vi "SetXL_CellValues_2D_Dbl.vi"(0 "Refnum Cluster In":T1, 5 "Start":cluster{"Column":i32, "Row":i32}, 9 "data":dbl[][](array[numeric]), 11 "error in":errorcluster) -> (4 "Refnum Cluster Out":T1, 15 "error out":errorcluster)   [LabVIEW 2017, in "excel_configuration.lvlib"]
uses:
  excel_configuration.lvlib
  858a33e0-4cb3-45c4-8fa4-0a07d001454b.vi
  <vilib>/Utility/error.llb/Clear Errors.vi
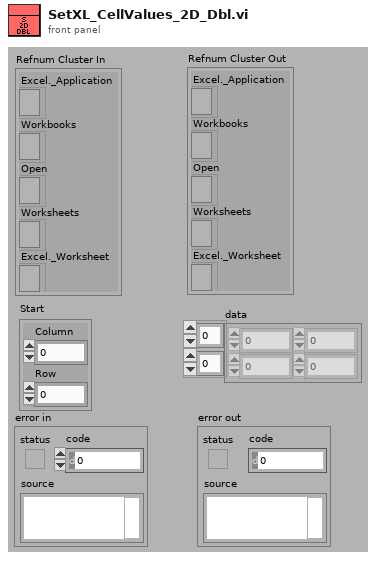
[diagram p1: front panel]
types:
  T1 = cluster{"Excel._Application":refnum<k7>, "Workbooks":refnum<k7>, "Open":refnum<k7>, "Worksheets":refnum<k7>, "Excel._Worksheet":refnum<k7>}
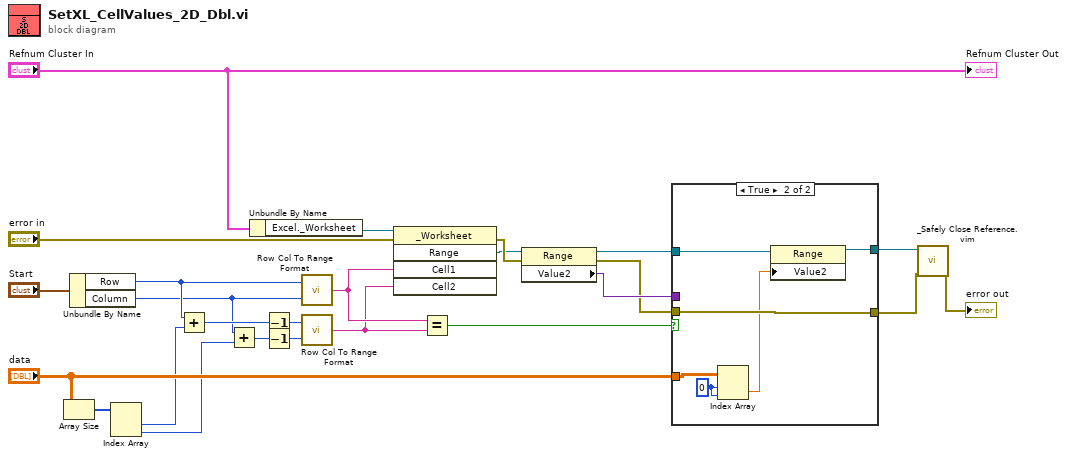
[diagram p0: block diagram]
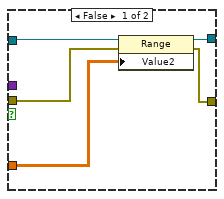
[diagram p2: hidden frame]
diagram:
  n1 = Array Size(array="data") -> (size(s)=w9:i32[])
  n2 = Unbundle By Name("Start") -> ("Row"=w8:i32, "Column"=w3:i32)
  n3 = Index Array(array=w9) -> (element #1=w5:i32, element #2=w4:i32)  [unwired: 2 in]
  n4 = Add(x=w8, y=w5) -> (x+y=w6:i32)
  n5 = Add(x=w3, y=w4) -> (x+y=w7:i32)
  n6 = Unbundle By Name("Refnum Cluster In") -> ("Excel._Worksheet"=w17:refnum<k7>)
  n7 = Decrement(x=w6) -> (x-1=w1:i32)
  n8 = Decrement(x=w7) -> (x-1=w2:i32)
  n9 = call "Row Col To Range Format.vi"("Column"=w3, "Row"=w8) -> ("Output String"=w20:string)
  n10 = call "Row Col To Range Format.vi"("Column"=w2, "Row"=w1) -> ("Output String"=w19:string)
  n11 = invoke class="_Worksheet" method="Range"(reference=w17, error in="error in", "Cell1"=w20, "Cell2"=w19) -> (error out=w24:errorcluster, "Range"=w23:refnum<k7>)  [unwired: 1 in, 3 out]
  n12 = Equal?(x=w20, y=w19) -> (x = y?=w18:bool)
  n13 = property class="Range"(reference=w23, error in=w24) -> (reference out=w14:refnum<k7>, error out=w15:errorcluster, "Value2"=w21:variant)
  n14 = case shown="True" w18 {
    tunnel: w21 -> [_ _]
    tunnel: [w27 w36] -> w12
    tunnel: w15 -> [w28 w36]
    tunnel: w14 -> [w30 w35]
    tunnel: [w29 w34] -> w13
    tunnel: "data" -> [w26 w33]
    frame False {
      n15 = property class="Range"(reference=w30, error in=w28, "Value2"=w26) -> (reference out=w29:refnum<k7>, error out=w27:errorcluster)
    }
    frame True {
      w32 = 0 ("index (row)")
      n16 = Index Array(array=w33, index (row)=w32, index (col)=w32) -> (element=w31:dbl)
      n17 = property class="Range"(reference=w35, "Value2"=w31) -> (reference out=w34:refnum<k7>)  [unwired: 1 in, 1 out]
    }
  }
  n18 = call "_Safely Close Reference.vim"("error in (no error)"=w12, "Automation Refnum in"=w13) -> ("error out"=→"error out":errorcluster)  [unwired: 9 in]
  "Refnum Cluster Out" <- "Refnum Cluster In"
